vi "Get Count.vi"(8 "error in (no error)":errorcluster caption="错误输入（无错误）", 11 "具体聚集 输入":refnum<class "具体聚集.lvclass"> caption="DNL_LabVIEW Object in") -> (0 "error out":errorcluster caption="错误输出", 1 "Count":i32, 3 "具体聚集 输出":refnum<class "具体聚集.lvclass"> caption="DNL_LabVIEW Object out")   [LabVIEW 2011, in "迭代器.lvlib" / "具体聚集.lvclass"]
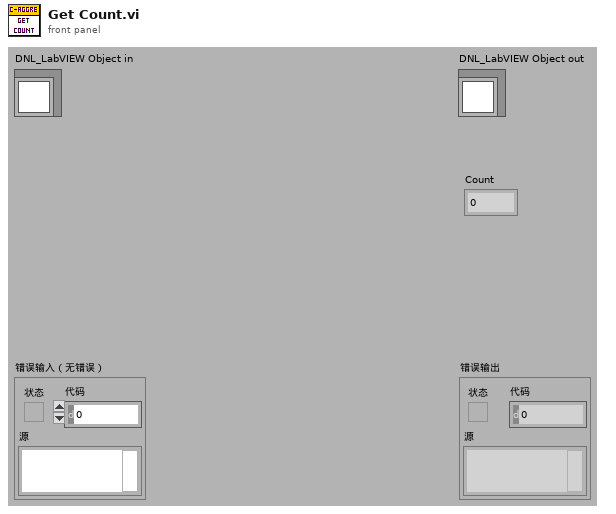
[diagram p1: front panel]
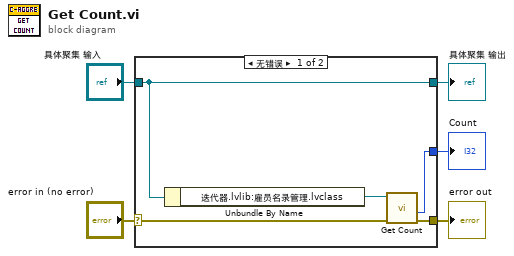
[diagram p0: block diagram]
diagram:
  n1 = case shown="无错误" "error in (no error)" {
    selector: "error in (no error)" -> [w8 w12]
    tunnel: [w7 w12] -> w4
    tunnel: [w10 w11] -> w2
    tunnel: "具体聚集 输入" -> [w10 w11]
    tunnel: [w6 _] -> w1
    frame No Error {
      n2 = Unbundle By Name(w10) -> ("迭代器.lvlib:雇员名录管理.lvclass"=w9:refnum<class "雇员名录管理.lvclass">)
      n3 = call "Get Count.vi"("error in (no error)"=w8, "雇员名录管理 输入"=w9) -> ("error out"=w7:errorcluster, "Count"=w6:i32)  [unwired: 7 in, 1 out]
    }
    frame Error {
    }
  }
  "error out" <- w4
  "具体聚集 输出" <- w2
  "Count" <- w1
